vi "K24xx_OpAmp_meas_2.vi"(7 "S1":bool, 8 "K24xx error in":errorcluster, 9 "S2":bool, 11 "K24xx VISA in":refnum<visa-resource-name>) -> (1 "K24xx error out":errorcluster, 3 "K24xx VISA out":refnum<visa-resource-name>, 5 "Out DUT1":dbl)   [LabVIEW 2014]
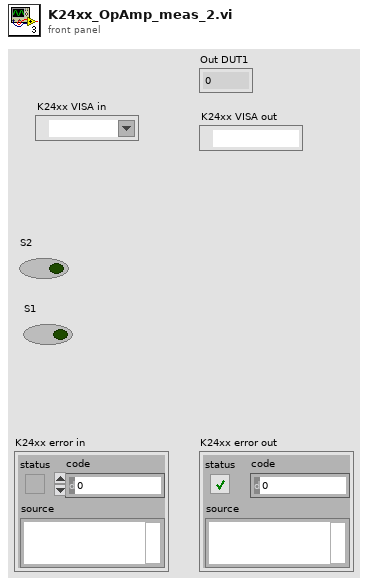
[diagram p1: front panel]
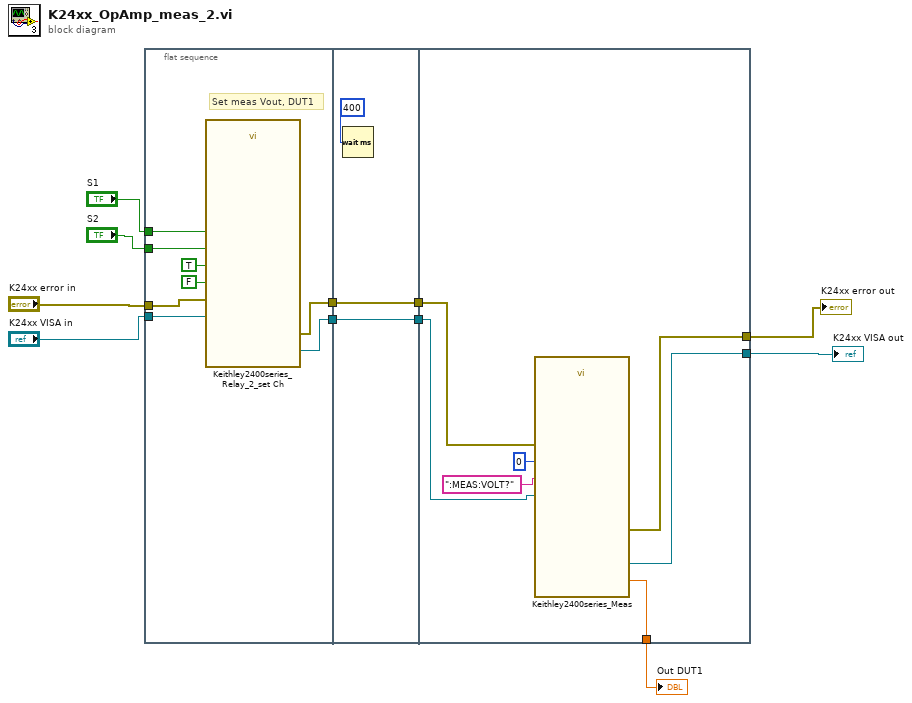
[diagram p0: block diagram]
diagram:
  n1 = flat-sequence {
    tunnel: "S1" -> [w19]
    tunnel: "S2" -> [w18]
    tunnel: "K24xx error in" -> [w17]
    tunnel: "K24xx VISA in" -> [w16]
    tunnel: [w13] -> w11
    tunnel: [w12] -> w10
    tunnel: w11 -> [w21]
    tunnel: [w21] -> w9
    tunnel: w10 -> [w20]
    tunnel: [w20] -> w8
    tunnel: [w24] -> w6
    tunnel: [w23] -> w7
    tunnel: w9 -> [w26]
    tunnel: w8 -> [w25]
    tunnel: [w28] -> w1
    frame #0 {
      # "Set meas Vout, DUT1"
      n2 = call "Keithley2400series_Relay_2_set Ch.vi"("Ch4"=FALSE, "Ch1"=w19, "error in (no error)"=w17, "Ch3"=TRUE, "Ch2"=w18, "VISA Refnum in"=w16) -> ("error out"=w12:errorcluster, "VISA Refnum out"=w13:refnum<visa-resource-name>)  [unwired: 4 in]
    }
    frame #1 {
      n3 = Wait (ms)(milliseconds to wait=u32 400) -> ()  [unwired: 1 out]
    }
    frame #2 {
      n4 = call "Keithley2400series_Meas.vi"("MEAS:<f>"=":MEAS:VOLT?", "error in (no error)"=w25, "MEAS mode, 0 Volt"=u16 0, "VISA resource name in"=w26) -> ("error out"=w24:errorcluster, "Замер"=w28:dbl, "VISA out"=w23:refnum<visa-resource-name>)  [unwired: 1 in, 1 out]
    }
  }
  "Out DUT1" <- w1
  "K24xx error out" <- w6
  "K24xx VISA out" <- w7
